vi "Scan Barcode.vi"(0 "Operator":string, 11 "error in":errorcluster) -> (4 "Operator Name Out":string, 6 "Serial Number Out":string, 8 "Cancelled?":bool, 15 "error out":errorcluster)   [LabVIEW 2024]
doc: "User inputs name and serial number to log with results. Username persists between subsequent test."
uses:
  <vilib>/addons/_JKI Toolkits/State Machine/_JKI_lib_State_Machine.llb/Select State(s)_err__jki_lib_state_machine.vi
  <vilib>/addons/_JKI Toolkits/State Machine/_JKI_lib_State_Machine.llb/Periodic Trigger__ogtk__JKI-SM__jki_lib_state_machine.vi
  <userlib>/_OpenG.lib/appcontrol/appcontrol.llb/openg_application_control.lvlib
  <userlib>/_OpenG.lib/time/time.llb/openg_time.lvlib
panel:
  in  "OK":bool
  in  "Cancel":bool
  in  "Serial Number":string
  # "SCAN BARCODE"
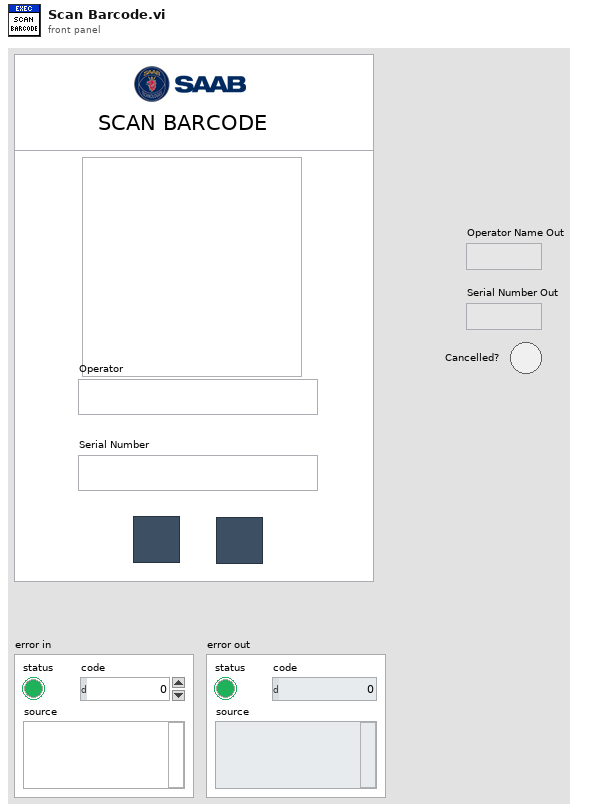
[diagram p1: front panel]
types:
  T1 = enum32{"Invalid", "Standard", "Closed", "Hidden", "Minimized", "Maximized"}
  T2 = enum32{"invalid app kind", "Development System", "Run Time System", "Student Edition", "Embedded LabVIEW", "Evaluation", "Custom"}
  T3 = cluster{"Core":cluster{"Current VI Reference":refnum<vi>, "Close Panel on Exit?":bool}, "Operator":string, "Serial Number":string}
  T4 = cluster{"Current VI Reference":refnum<vi>, "Close Panel on Exit?":bool}
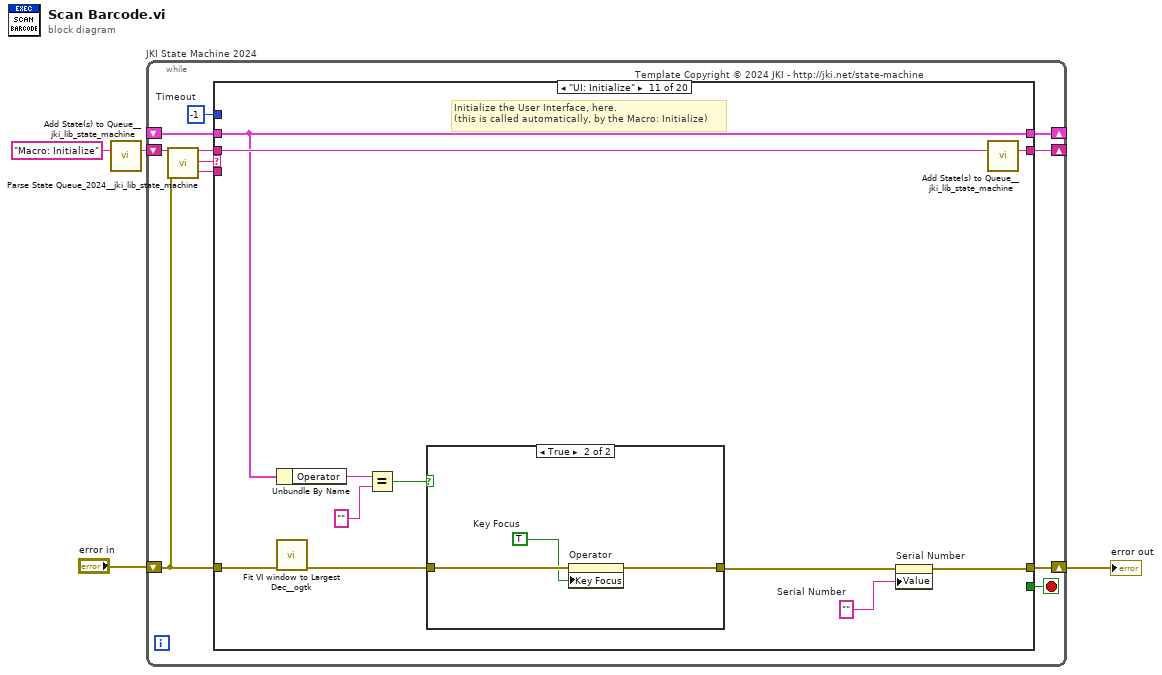
[diagram p0: block diagram]
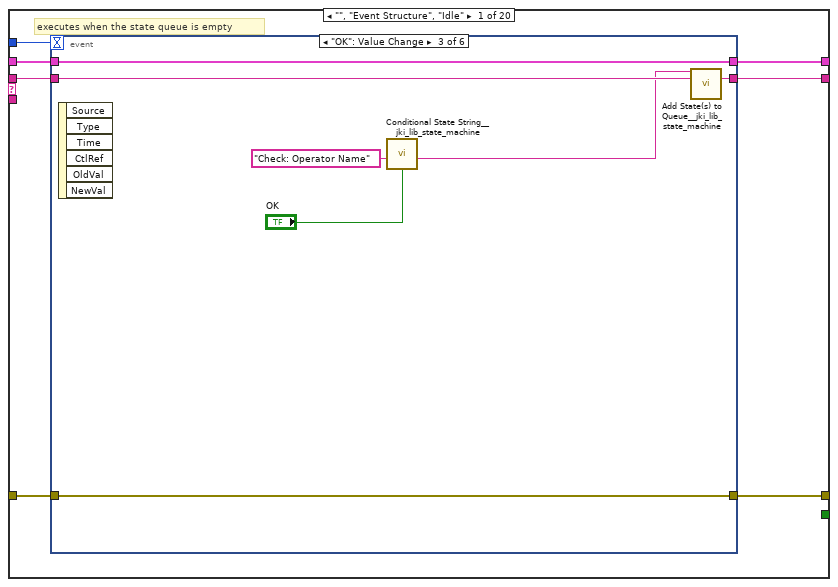
[diagram p2: hidden frame]
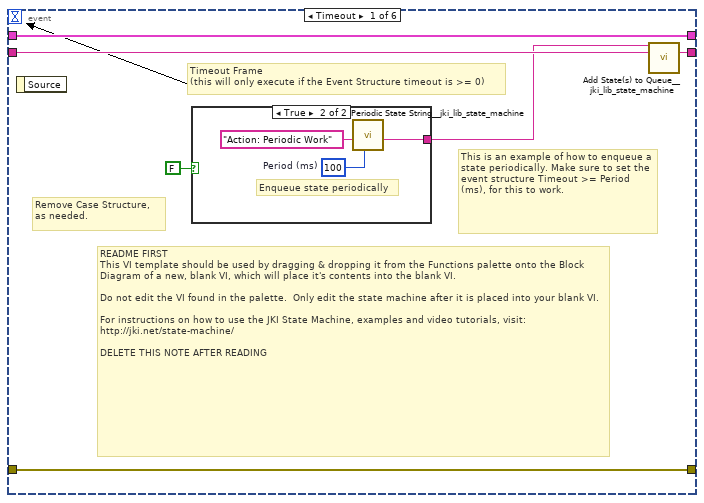
[diagram p3: hidden frame]
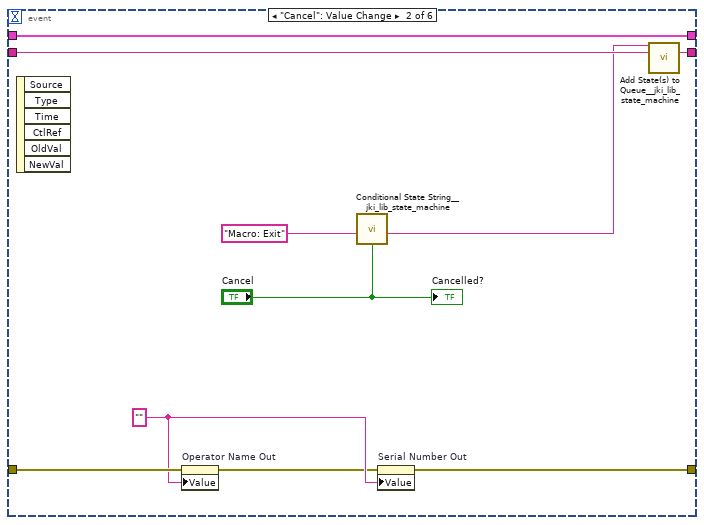
[diagram p5: hidden frame]
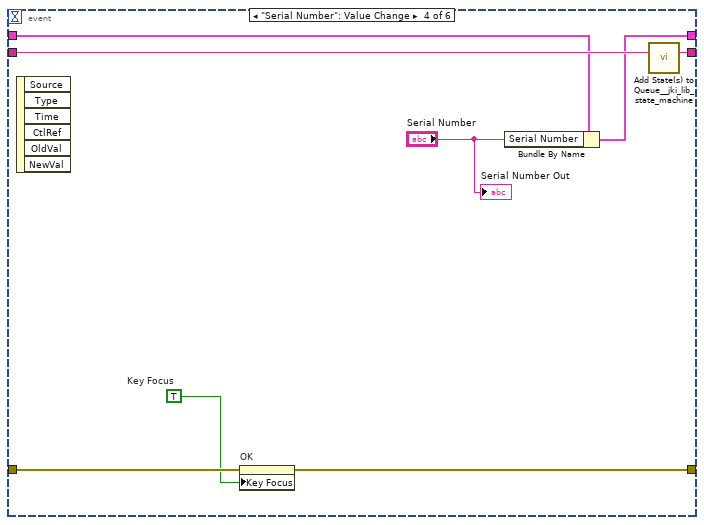
[diagram p6: hidden frame]
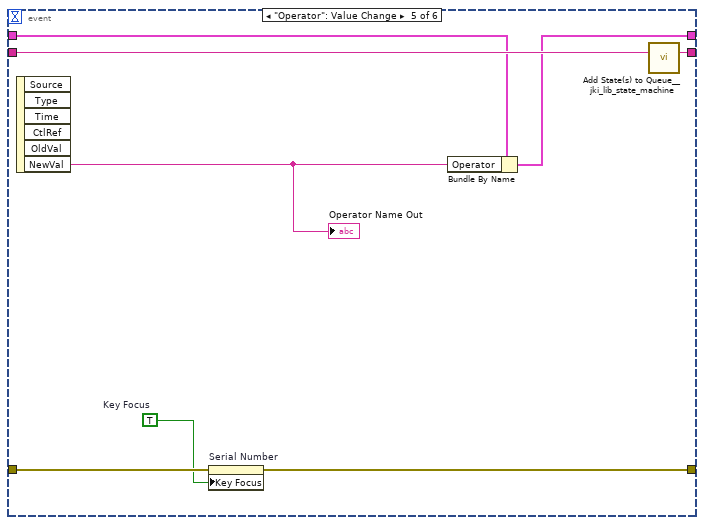
[diagram p7: hidden frame]
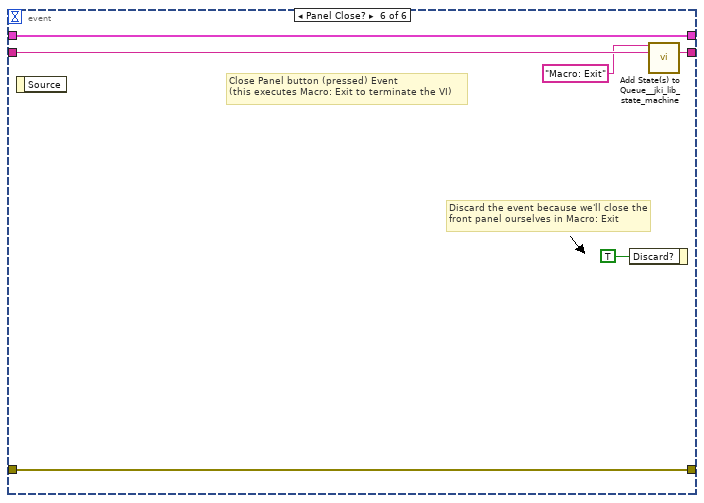
[diagram p8: hidden frame]
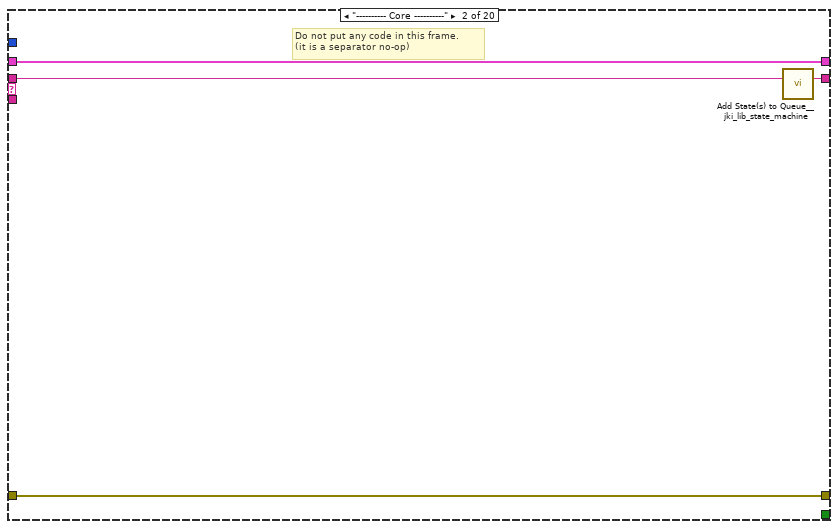
[diagram p9: hidden frame]
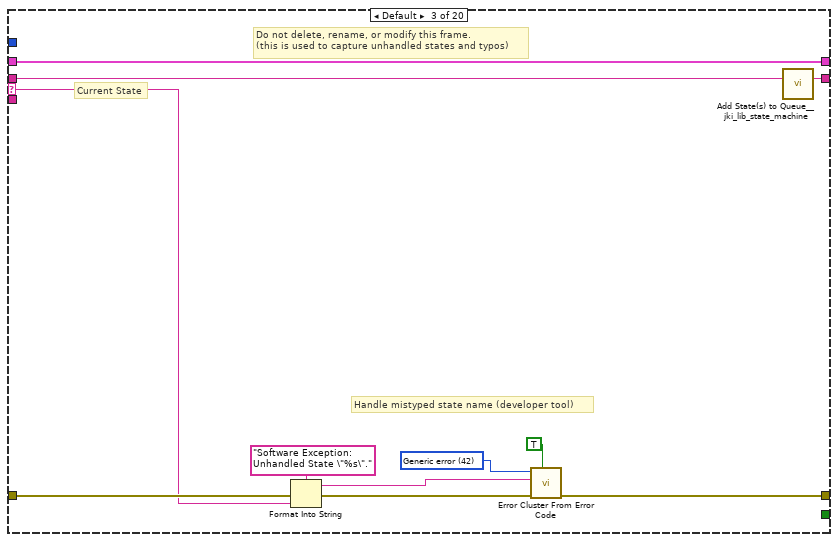
[diagram p10: hidden frame]
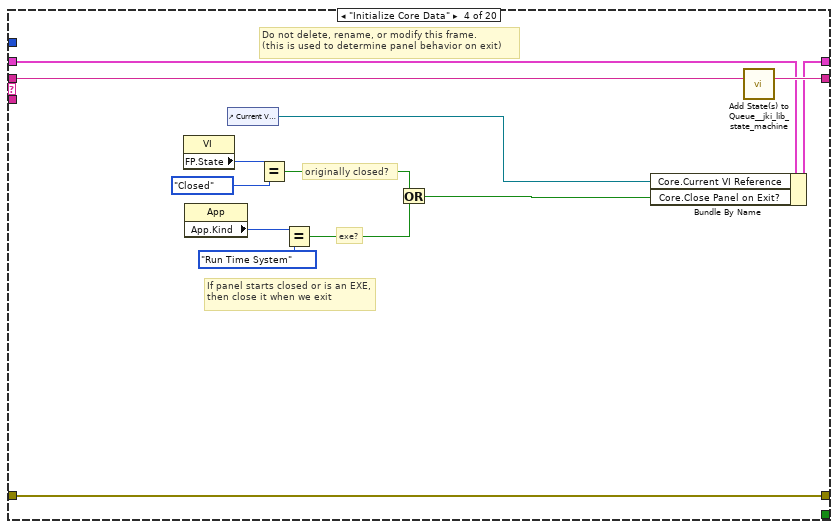
[diagram p11: hidden frame]
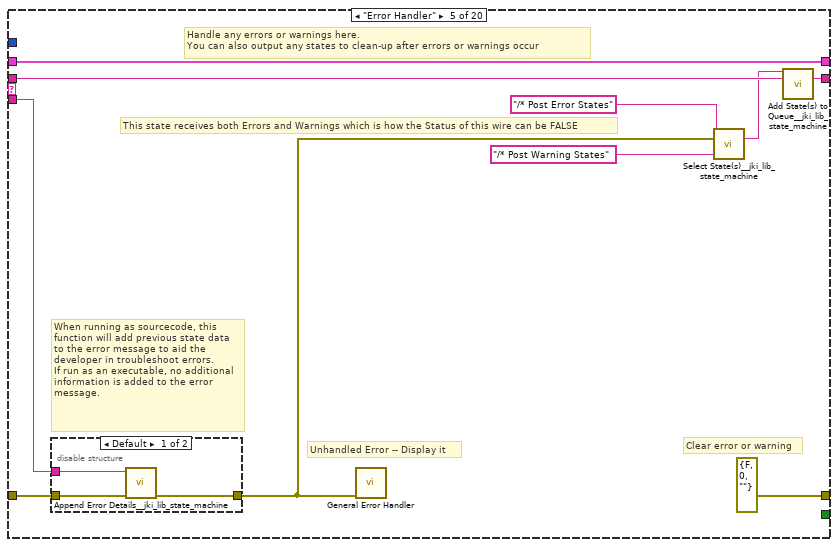
[diagram p12: hidden frame]
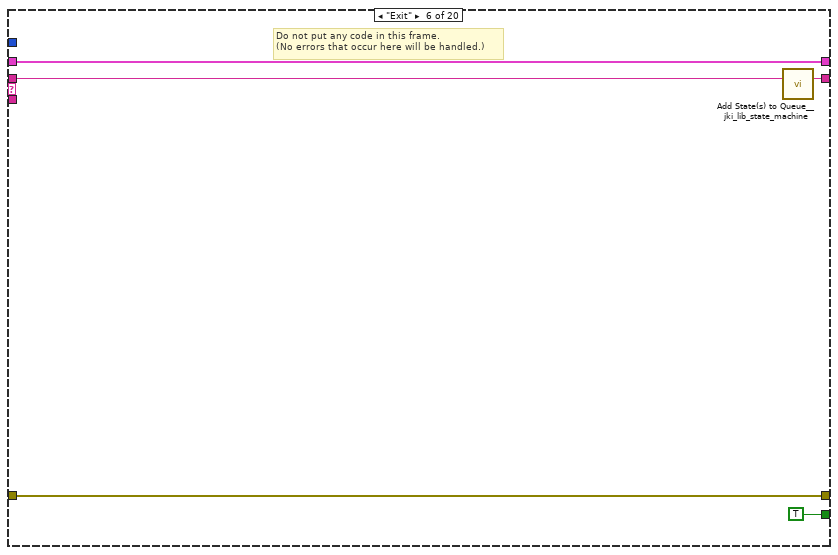
[diagram p14: hidden frame]
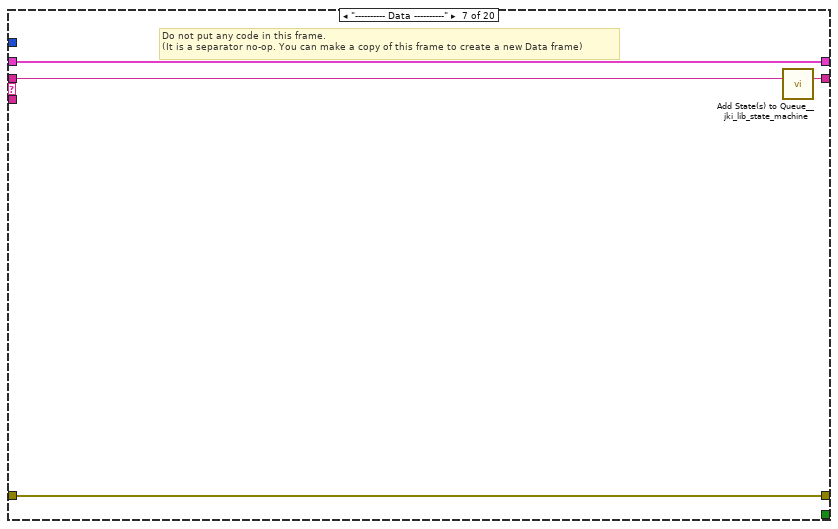
[diagram p15: hidden frame]
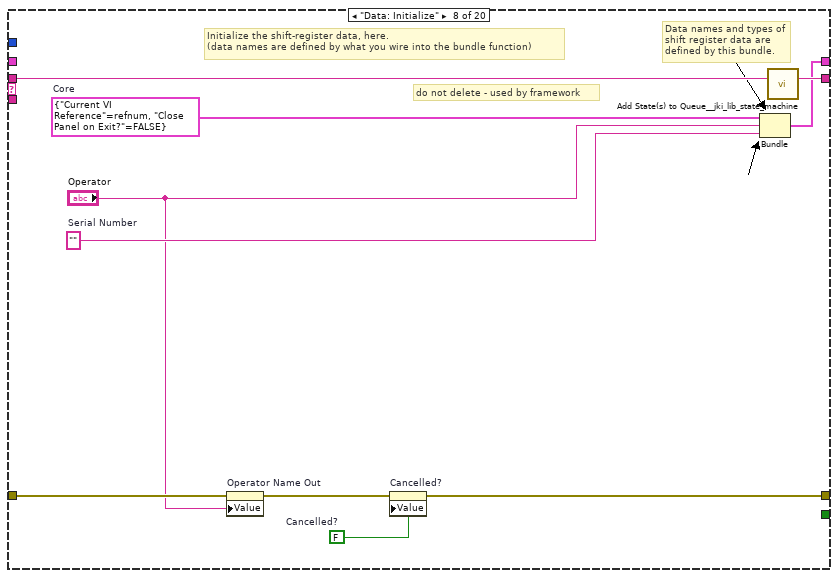
[diagram p16: hidden frame]
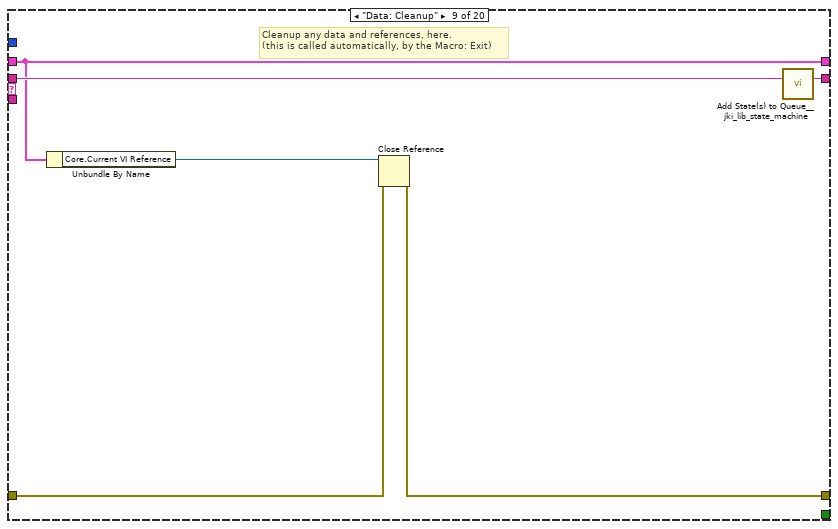
[diagram p17: hidden frame]
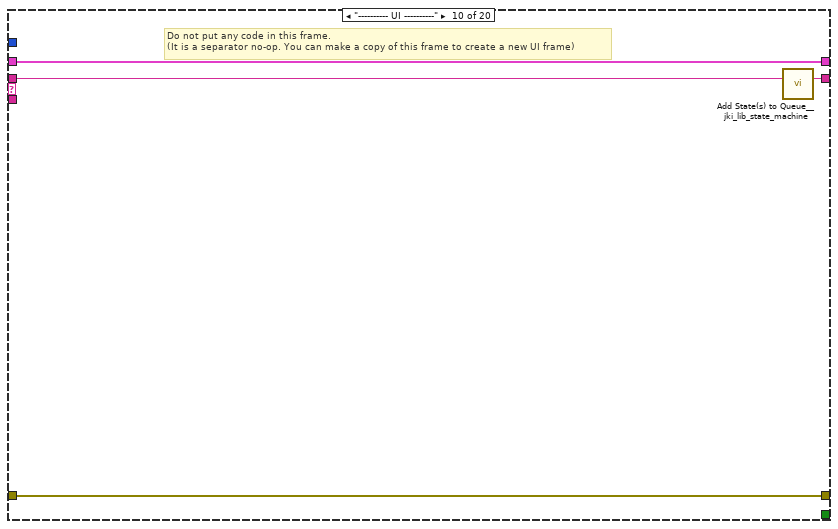
[diagram p18: hidden frame]
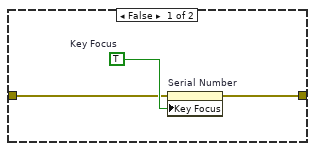
[diagram p19: hidden frame]
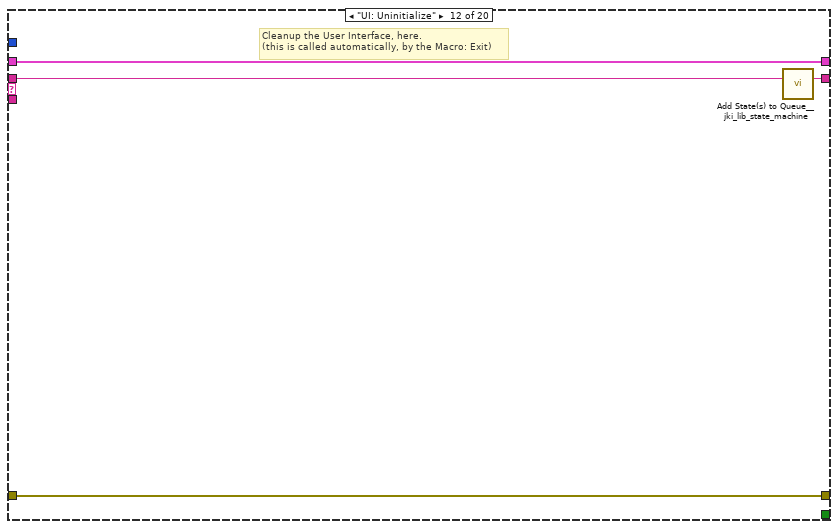
[diagram p20: hidden frame]
diagram:
  n1 = call <vilib>:"Add State(s) to Queue__jki_lib_state_machine.vi"("State(s) in (\"\")"="Macro: Initialize") -> ("States Out"=w4:string)  [unwired: 14 in]
  n2 = while "JKI State Machine 2024" {
    shift-right: [w8] -> _
    shift-left: _ -> [w7]
    shift-right: [w11] -> w1
    shift-left: "error in" -> [w5]
    shift-right: [w10] -> _
    shift-left: w4 -> [w12]
    stop <- w9 stop-if-true
    w6 = -1  # Timeout
    # "Template Copyright © 2024 JKI - http://jki.net/state-machine"
    n3 = call <vilib>:"Parse State Queue_2024__jki_lib_state_machine.vi"("State Queue"=w12, "Error In (no error)"=w5) -> ("Remaining States"=w14:string, "Current State"=w15:string, "Arguments"=w13:string)  [unwired: 11 in]
    n4 = case shown="\"UI: Initialize\"" w15 {
      selector: w15 -> [_ _ w75 _ _ _ _ _ _ _ _ _ _ _ _ _ _ _ _ _]
      tunnel: w14 -> [w22 w74 w79 w98 w108 w117 w121 w131 w137 w141 w152 w162 w168 w179 w248 w253 w262 w266 w275 w297]
      tunnel: w13 -> [_ _ _ _ w103 _ _ _ _ _ _ _ w163 w173 _ _ _ _ _ _]
      tunnel: w7 -> [w20 w71 w77 w91 w105 w115 w118 _ w132 w138 w148 w160 w166 w175 w245 w250 w260 w263 w269 w290]
      tunnel: [w19 w72 w81 w95 errorcluster {"status"=FALSE, "code"=0, "source"=""} ("error out") w114 w119 w123 w133 w139 w144 w159 w164 w176 w246 w251 w257 w264 w267 w291] -> w11
      tunnel: w5 -> [w16 w72 w80 w95 w104 w114 w119 w126 w134 w139 w149 w159 w165 w177 w246 w251 w257 w264 w270 w292]
      tunnel: [w21 w73 w78 w97 w107 w116 w120 w130 w136 w140 w151 w161 w167 w178 w247 w252 w261 w265 w274 w296] -> w10
      tunnel: [_ _ _ _ _ TRUE _ _ _ _ _ _ _ _ _ _ _ _ _ _] -> w9
      tunnel: [w18 w71 w77 w96 w105 w115 w118 w129 w132 w138 w148 w160 w166 w175 w245 w250 w260 w263 w269 w290] -> w8
      tunnel: w6 -> [w17 _ _ _ _ _ _ _ _ _ _ _ _ _ _ _ _ _ _ _]
      frame "", "Event Structure", "Idle" {
        # "executes when the state queue is empty"
        n5 = event shown="[2] \"OK\": Value Change" {
          selector: _ -> [_ _ _ _ _ _]
          dyn-events: _ -> [_ _ _ _ _ _]
          timeout: w17 -> [_ _ _ _ _ _]
          tunnel: w22 -> [w28 w41 w48 w56 w64 w70]
          tunnel: [w27 w40 w47 w55 w63 w69] -> w21
          tunnel: w20 -> [w25 w36 w45 w54 w62 w67]
          tunnel: [w26 w32 w46 w50 w59 w68] -> w19
          tunnel: w16 -> [w26 w35 w46 w51 w58 w68]
          tunnel: [w25 w36 w45 w53 w61 w67] -> w18
          event Timeout {
            # "Remove Case Structure, as needed."
            # "This is an example of how to enqueue a state periodically. Make sure to set the event structure Timeout >= Period (ms), for this to work."
            # "README FIRST\nThis VI template should be used by dragging & dropping it from the Functions palette onto the Block Diagram of a new, blank VI, which will place it's contents into the blank VI.\n\nDo not edit the VI found in the palette.  Only edit the state machine after it is placed into your blank VI.\n\nFor instructions on how to use the JKI State Machine, examples and video tutorials, visit:\nhttp://jki.net/state-machine/\n\nDELETE THIS NOTE AFTER READING"
            # "Timeout Frame\n(this will only execute if the Event Structure timeout is >= 0)"
            n6 = event-data() -> ()  [unwired: 1 in, 1 out]
            n7 = case shown="True" FALSE {
              tunnel: [_ w31] -> w24
              frame False {
              }
              frame True {
                w29 = u32 100  # Period (ms)
                # "Enqueue state periodically"
                n8 = call <vilib>:"Periodic State String__jki_lib_state_machine.vi"("Period (ms)"=w29, "State"="Action: Periodic Work") -> ("State Out"=w31:string)  [unwired: 9 in]
              }
            }
            n9 = call <vilib>:"Add State(s) to Queue__jki_lib_state_machine.vi"("State(s) in Front (\"\")"=w24, "State(s) in (\"\")"=w28) -> ("States Out"=w27:string)  [unwired: 13 in]
          }
          event "Cancel": Value Change {
            w34 = ""
            n10 = event-data() -> ()  [unwired: 1 in, 6 out]
            n11 = property on="Operator Name Out" class="Str"(error in=w35, "Value"=w34) -> (error out=w33:errorcluster)  [unwired: 1 in, 1 out]
            n12 = call <vilib>:"Conditional State String__jki_lib_state_machine.vi"("Do State(s)?"="Cancel", "State"="Macro: Exit") -> ("State Out"=w38:string)  [unwired: 7 in]
            n13 = property on="Serial Number Out" class="Str"(error in=w33, "Value"=w34) -> (error out=w32:errorcluster)  [unwired: 1 in, 1 out]
            n14 = call <vilib>:"Add State(s) to Queue__jki_lib_state_machine.vi"("State(s) in Front (\"\")"=w38, "State(s) in (\"\")"=w41) -> ("States Out"=w40:string)  [unwired: 13 in]
            "Cancelled?" <- "Cancel"
          }
          event "OK": Value Change {
            n15 = event-data() -> ()  [unwired: 1 in, 6 out]
            n16 = call <vilib>:"Conditional State String__jki_lib_state_machine.vi"("Do State(s)?"="OK", "State"="Check: Operator Name") -> ("State Out"=w43:string)  [unwired: 7 in]
            n17 = call <vilib>:"Add State(s) to Queue__jki_lib_state_machine.vi"("State(s) in Front (\"\")"=w43, "State(s) in (\"\")"=w48) -> ("States Out"=w47:string)  [unwired: 13 in]
          }
          event "Serial Number": Value Change {
            w49 = TRUE  # Key Focus
            n18 = event-data() -> ()  [unwired: 1 in, 6 out]
            n19 = property on="OK" class="Bool"(error in=w51, "Key Focus"=w49) -> (error out=w50:errorcluster)  [unwired: 1 in, 1 out]
            n20 = Bundle By Name(cluster=w54, "Serial Number"="Serial Number") -> (w53:T3)
            n21 = call <vilib>:"Add State(s) to Queue__jki_lib_state_machine.vi"("State(s) in (\"\")"=w56) -> ("States Out"=w55:string)  [unwired: 14 in]
            "Serial Number Out" <- "Serial Number"
          }
          event "Operator": Value Change {
            w57 = TRUE  # Key Focus
            n22 = event-data() -> ("NewVal"=w60:string)  [unwired: 1 in, 5 out]
            "Operator Name Out" <- w60
            n23 = property on="Serial Number" class="Str"(error in=w58, "Key Focus"=w57) -> (error out=w59:errorcluster)  [unwired: 1 in, 1 out]
            n24 = Bundle By Name(cluster=w62, "Operator"=w60) -> (w61:T3)
            n25 = call <vilib>:"Add State(s) to Queue__jki_lib_state_machine.vi"("State(s) in (\"\")"=w64) -> ("States Out"=w63:string)  [unwired: 14 in]
          }
          event Panel Close? {
            # "Discard the event because we'll close the front panel ourselves in Macro: Exit"
            # "Close Panel button (pressed) Event\n(this executes Macro: Exit to terminate the VI)"
            n26 = event-data() -> ()  [unwired: 1 in, 1 out]
            n27 = event-data("Discard?"=TRUE) -> ()  [unwired: 1 in, 1 out]
            n28 = call <vilib>:"Add State(s) to Queue__jki_lib_state_machine.vi"("State(s) in Front (\"\")"="Macro: Exit", "State(s) in (\"\")"=w70) -> ("States Out"=w69:string)  [unwired: 13 in]
          }
        }
      }
      frame "---------- Core ----------" {
        # "Do not put any code in this frame.\n(it is a separator no-op)"
        n29 = call <vilib>:"Add State(s) to Queue__jki_lib_state_machine.vi"("State(s) in (\"\")"=w74) -> ("States Out"=w73:string)  [unwired: 14 in]
      }
      frame Default {
        w84 = 42 items=["No error", "Argument error", "Memory is full", "Out of zone", "End of file", "File already open", "Generic file I/O error", "File not found", "File permission error", "Disk is full", "Duplicate path", "Too many files open", "System feature not enabled", "Resource file not found", "Cannot add resource", "Resource not found", "Image not found", "Image memory error", "Pen does not exist", "Config type invalid", "Config token not found", "Config parse error", "Config memory error", "Bad external code format", "Bad external code offset", "External code not present", "Null window", "Destroy window error", "Null menu", "Print aborted", "Bad print record", "Print driver error", "Windows error during printing", "Memory error during printing", "Print dialog error", "Generic print error", "Invalid device refnum", "Device not found", "Device parameter error", "Device unit error", "Cannot open device", "Device call aborted", "Generic error", "Cancelled by user", "Object ID too low", "Object ID too high", "Object not in heap", "Unknown heap", "Unknown object (invalid DefProc)", "Unknown object (DefProc not in table)", "Message out of range", "Invalid (null) method", "Unknown message", "Manager call not supported", "Bad address", "Network operation in progress", "Network operation timed out", "Connection is busy", "Network attribute not supported", "Network error", "Address in use", "System out of memory", "Connection aborted", "Connection refused", "Not connected", "Already connected", "Connection closed", "Initialization error (interapplication manager)", "Bad occurrence", "Wait on unbound occurrence handler", "Occurrence queue overflow", "Datalog type conflict", "Unused", "Unrecognized type (interapplication manager)", "Memory corrupt", "Failed to make temporary DLL", "Old CIN version", "Drag socket not found", "Failed to load drop-object", "Failed to register OLE object", "Failed to release OLE object", "Format specifier type mismatch", "Unknown format specifier", "Too few format specifiers", "Too many format specifiers", "Scan failed", "Newer CIN version", "Error converting to variant", "Runtime menu error", "Password tampered", "Variant attribute not found", "Incompatible variant data type", "Event data is not available", "Event Store is not present", "Occurrence is not found", "Event Queue is not created", "Event info is not available", "Refnum passed is NULL", "Error retrieving Class GUID", "Error retrieving CoClass GUID", "Error retrieving TypeLib GUID.", "Bad built application magic bytes.", "Specific driver is different from the specific driver associated with the Logical Name.", "There is no session opened to the class driver.", "Max Error", "MAX - Error with config objects", "MAX - Error loading configuration", "MAX - Group not supported"]
        # "Current State"
        # "Do not delete, rename, or modify this frame.\n(this is used to capture unhandled states and typos)"
        # "Handle mistyped state name (developer tool)"
        n30 = Format Into String(format string="Software Exception: Unhandled State \"%s\"." ("message"), error in=w80, w75) -> (resulting string=w83:string, error out=w82:errorcluster)  [unwired: 1 in]
        n31 = call <vilib>:"Error Cluster From Error Code.vi"("show call chain? (False)"=TRUE, "error in (no error)"=w82, "error message (\"\")"=w83, "error code (0)"=w84) -> ("error out"=w81:errorcluster)  [unwired: 5 in]
        n32 = call <vilib>:"Add State(s) to Queue__jki_lib_state_machine.vi"("State(s) in (\"\")"=w79) -> ("States Out"=w78:string)  [unwired: 14 in]
      }
      frame "Initialize Core Data" {
        # "Do not delete, rename, or modify this frame.\n(this is used to determine panel behavior on exit)"
        # "originally closed?"
        # "exe?"
        # "If panel starts closed or is an EXE, then close it when we exit"
        n33 = property class="VI"() -> ("FP.State"=w88:T1)  [unwired: 2 in, 2 out]
        n34 = property class="App"() -> ("App.Kind"=w94:T2)  [unwired: 2 in, 2 out]
        n35 = control-ref of="Current VI Reference"() -> (w89:refnum<vi>)
        n36 = Equal?(x=w88, y=T1."Closed" ("Front Panel Window:State")) -> (x = y?=w86:bool)
        n37 = Equal?(x=w94, y=T2."Run Time System" ("Application:Kind")) -> (x = y?=w92:bool)
        n38 = Or(x=w86, y=w92) -> (x .or. y?=w90:bool)
        n39 = Bundle By Name(cluster=w91, "Core.Current VI Reference"=w89, "Core.Close Panel on Exit?"=w90) -> (w96:T3)
        n40 = call <vilib>:"Add State(s) to Queue__jki_lib_state_machine.vi"("State(s) in (\"\")"=w98) -> ("States Out"=w97:string)  [unwired: 14 in]
      }
      frame "Error Handler" {
        # "When running as sourcecode, this function will add previous state data to the error message to aid the developer in troubleshoot errors.\nIf run as an executable, no additional information is added to the error message."
        # "This state receives both Errors and Warnings which is how the Status of this wire can be FALSE"
        # "Unhandled Error -- Display it"
        # "Handle any errors or warnings here.\nYou can also output any states to clean-up after errors or warnings occur"
        # "Clear error or warning"
        n41 = disable-structure shown="Default" {
          disable-tunnel: w104 -> [w111 w112]
          disable-tunnel: w103 -> [w110 _]
          disable-tunnel: [w109 w112] -> w102
          frame condition #0 (active) {
            n42 = call <vilib>:"Append Error Details__jki_lib_state_machine.vi"("error in (no error)"=w111, "Previous State and Argument(s)"=w110) -> ("error out"=w109:errorcluster)  [unwired: 9 in]
          }
          frame condition #1 {
          }
        }
        n43 = call <vilib>:"General Error Handler.vi"("error in (no error)"=w102) -> ()  [unwired: 10 in, 5 out]
        n44 = call-poly <vilib>:"Select State(s)__jki_lib_state_machine.vi"("State(s) if True (\"\")"="/* Post Error States", "Select"=w102, "State(s) if False (\"\")"="/* Post Warning States") -> ("States Out"=w100:string)  [unwired: 12 in]
        n45 = call <vilib>:"Add State(s) to Queue__jki_lib_state_machine.vi"("State(s) in Front (\"\")"=w100, "State(s) in (\"\")"=w108) -> ("States Out"=w107:string)  [unwired: 13 in]
      }
      frame "Exit" {
        # "Do not put any code in this frame.\n(No errors that occur here will be handled.)"
        n46 = call <vilib>:"Add State(s) to Queue__jki_lib_state_machine.vi"("State(s) in (\"\")"=w117) -> ("States Out"=w116:string)  [unwired: 14 in]
      }
      frame "---------- Data ----------" {
        # "Do not put any code in this frame.\n(It is a separator no-op. You can make a copy of this frame to create a new Data frame)"
        n47 = call <vilib>:"Add State(s) to Queue__jki_lib_state_machine.vi"("State(s) in (\"\")"=w121) -> ("States Out"=w120:string)  [unwired: 14 in]
      }
      frame "Data: Initialize" {
        w122 = FALSE  # Cancelled?
        w127 = T4 {"Current VI Reference"=refnum, "Close Panel on Exit?"=FALSE}  # Core
        w128 = ""  # Serial Number
        # "do not delete - used by framework"
        # "Data names and types of shift register data are defined by this bundle."
        # "Initialize the shift-register data, here.\n(data names are defined by what you wire into the bundle function)"
        n48 = property on="Operator Name Out" class="Str"(error in=w126, "Value"="Operator") -> (error out=w124:errorcluster)  [unwired: 1 in, 1 out]
        n49 = property on="Cancelled?" class="Bool (strict)"(error in=w124, "Value"=w122) -> (error out=w123:errorcluster)  [unwired: 1 in, 1 out]
        n50 = Bundle("Core"=w127, "Operator"="Operator", "Serial Number"=w128) -> (w129:T3)  [unwired: 1 in]
        n51 = call <vilib>:"Add State(s) to Queue__jki_lib_state_machine.vi"("State(s) in (\"\")"=w131) -> ("States Out"=w130:string)  [unwired: 14 in]
      }
      frame "Data: Cleanup" {
        # "Cleanup any data and references, here.\n(this is called automatically, by the Macro: Exit)"
        n52 = Unbundle By Name(w132) -> ("Core.Current VI Reference"=w135:refnum<vi>)
        n53 = Close Reference(reference=w135, error in (no error)=w134) -> (error out=w133:errorcluster)
        n54 = call <vilib>:"Add State(s) to Queue__jki_lib_state_machine.vi"("State(s) in (\"\")"=w137) -> ("States Out"=w136:string)  [unwired: 14 in]
      }
      frame "---------- UI ----------" {
        # "Do not put any code in this frame.\n(It is a separator no-op. You can make a copy of this frame to create a new UI frame)"
        n55 = call <vilib>:"Add State(s) to Queue__jki_lib_state_machine.vi"("State(s) in (\"\")"=w141) -> ("States Out"=w140:string)  [unwired: 14 in]
      }
      frame "UI: Initialize" {
        w142 = ""  # Serial Number
        # "Initialize the User Interface, here.\n(this is called automatically, by the Macro: Initialize)"
        n56 = Unbundle By Name(w148) -> ("Operator"=w147:string)
        n57 = call <userlib>:"Fit VI window to Largest Dec__ogtk.vi"("error in (no error)"=w149) -> ("error out"=w150:errorcluster)  [unwired: 5 in, 1 out]
        n58 = Equal?(x=w147, y="") -> (x = y?=w145:bool)
        n59 = case shown="True" w145 {
          tunnel: [w154 w157] -> w143
          tunnel: w150 -> [w153 w158]
          frame False {
            w155 = TRUE  # Key Focus
            n60 = property on="Serial Number" class="Str"(error in=w153, "Key Focus"=w155) -> (error out=w154:errorcluster)  [unwired: 1 in, 1 out]
          }
          frame True {
            w156 = TRUE  # Key Focus
            n61 = property on="Operator" class="Str"(error in=w158, "Key Focus"=w156) -> (error out=w157:errorcluster)  [unwired: 1 in, 1 out]
          }
        }
        n62 = property on="Serial Number" class="Str"(error in=w143, "Value"=w142) -> (error out=w144:errorcluster)  [unwired: 1 in, 1 out]
        n63 = call <vilib>:"Add State(s) to Queue__jki_lib_state_machine.vi"("State(s) in (\"\")"=w152) -> ("States Out"=w151:string)  [unwired: 14 in]
      }
      frame "UI: Uninitialize" {
        # "Cleanup the User Interface, here.\n(this is called automatically, by the Macro: Exit)"
        n64 = call <vilib>:"Add State(s) to Queue__jki_lib_state_machine.vi"("State(s) in (\"\")"=w162) -> ("States Out"=w161:string)  [unwired: 14 in]
      }
      frame "UI: Cursor Set" {
        # "Argument"
        # "Set and Unset Cursor Busy.\n(Usage: \"UI: Cursor Set >> Busy|Idle\")"
        n65 = case shown="\"Idle\", Default" w163 {
          tunnel: w165 -> [w170 w172]
          tunnel: [w169 w171] -> w164
          frame "Idle", Default {
            n66 = call <vilib>:"Unset Busy.vi"("error in (no error)"=w170) -> ("error out"=w169:errorcluster)  [unwired: 10 in]
          }
          frame "Busy" {
            n67 = call <vilib>:"Set Busy.vi"("error in (no error)"=w172) -> ("error out"=w171:errorcluster)  [unwired: 9 in, 1 out]
          }
        }
        n68 = call <vilib>:"Add State(s) to Queue__jki_lib_state_machine.vi"("State(s) in (\"\")"=w168) -> ("States Out"=w167:string)  [unwired: 14 in]
      }
      frame "UI: Front Panel State" {
        # "Argument"
        # "Set Front Panel Open or Closed\n(Usage: \"UI: Front Panel State >> Open|Close\")"
        n69 = Unbundle By Name(w175) -> ("Core.Current VI Reference"=w174:refnum<vi>)
        n70 = case shown="\"Minimize\", \"Minimized\"" w173 {
          tunnel: w177 -> [w185 w200 w211 w224 w237]
          tunnel: [w187 w201 w213 w226 w239] -> w176
          tunnel: w174 -> [w186 w198 w212 w225 w238]
          frame "Open", "Standard", Default {
            w180 = T1."Standard" ("State")
            n71 = property class="VI"(reference=w186, error in=w185) -> (reference out=w183:refnum<vi>, error out=w184:errorcluster, "FP.State"=w182:T1)
            n72 = Not Equal?(x=w182, y=w180) -> (x != y?=w181:bool)
            n73 = case shown="True" w181 {
              tunnel: [w191 w193] -> w187
              tunnel: w184 -> [w190 w193]
              tunnel: w183 -> [w189 _]
              tunnel: w180 -> [w188 _]
              frame True {
                n74 = invoke class="VI" method="FP.Open"(reference=w189, error in=w190, "Activate"=TRUE, "State"=w188) -> (error out=w191:errorcluster)  [unwired: 1 in, 4 out]
              }
              frame False {
              }
            }
          }
          frame "Close", "Closed" {
            n75 = property class="VI"(reference=w198, error in=w200) -> (reference out=w197:refnum<vi>, error out=w199:errorcluster, "FP.State"=w195:T1)
            n76 = Not Equal?(x=w195, y=T1."Closed" ("Front Panel Window:State")) -> (x != y?=w194:bool)
            n77 = case shown="True" w194 {
              tunnel: [w202 w205] -> w201
              tunnel: w199 -> [w202 w204]
              tunnel: w197 -> [_ w203]
              frame False {
              }
              frame True {
                n78 = invoke class="VI" method="FP.Close"(reference=w203, error in=w204) -> (error out=w205:errorcluster)  [unwired: 1 in, 2 out]
              }
            }
          }
          frame "Hidden", "Hide" {
            w206 = T1."Hidden" ("State")
            n79 = property class="VI"(reference=w212, error in=w211) -> (reference out=w209:refnum<vi>, error out=w210:errorcluster, "FP.State"=w208:T1)
            n80 = Not Equal?(x=w208, y=w206) -> (x != y?=w207:bool)
            n81 = case shown="True" w207 {
              tunnel: [w217 w218] -> w213
              tunnel: w210 -> [w216 w218]
              tunnel: w209 -> [w215 _]
              tunnel: w206 -> [w214 _]
              frame True {
                n82 = invoke class="VI" method="FP.Open"(reference=w215, error in=w216, "State"=w214) -> (error out=w217:errorcluster)  [unwired: 2 in, 4 out]
              }
              frame False {
              }
            }
          }
          frame "Minimize", "Minimized" {
            w219 = T1."Minimized" ("State")
            n83 = property class="VI"(reference=w225, error in=w224) -> (reference out=w222:refnum<vi>, error out=w223:errorcluster, "FP.State"=w221:T1)
            n84 = Not Equal?(x=w221, y=w219) -> (x != y?=w220:bool)
            n85 = case shown="True" w220 {
              tunnel: [w230 w231] -> w226
              tunnel: w223 -> [w229 w231]
              tunnel: w222 -> [w228 _]
              tunnel: w219 -> [w227 _]
              frame True {
                n86 = invoke class="VI" method="FP.Open"(reference=w228, error in=w229, "State"=w227) -> (error out=w230:errorcluster)  [unwired: 2 in, 4 out]
              }
              frame False {
              }
            }
          }
          frame "Maximize", "Maximized" {
            w232 = T1."Maximized" ("State")
            n87 = property class="VI"(reference=w238, error in=w237) -> (reference out=w235:refnum<vi>, error out=w236:errorcluster, "FP.State"=w234:T1)
            n88 = Not Equal?(x=w234, y=w232) -> (x != y?=w233:bool)
            n89 = case shown="True" w233 {
              tunnel: [w243 w244] -> w239
              tunnel: w236 -> [w242 w244]
              tunnel: w235 -> [w241 _]
              tunnel: w232 -> [w240 _]
              frame True {
                n90 = invoke class="VI" method="FP.Open"(reference=w241, error in=w242, "State"=w240) -> (error out=w243:errorcluster)  [unwired: 2 in, 4 out]
              }
              frame False {
              }
            }
          }
        }
        n91 = call <vilib>:"Add State(s) to Queue__jki_lib_state_machine.vi"("State(s) in (\"\")"=w179) -> ("States Out"=w178:string)  [unwired: 14 in]
      }
      frame "---------- Macro ----------" {
        # "Do not put any code in this frame.\n(It is a separator no-op. You can make a copy of this frame to create a new Macro frame)"
        n92 = call <vilib>:"Add State(s) to Queue__jki_lib_state_machine.vi"("State(s) in (\"\")"=w248) -> ("States Out"=w247:string)  [unwired: 14 in]
      }
      frame "Macro: Initialize" {
        w249 = "Data: Initialize\nInitialize Core Data\nUI: Initialize\nUI: Front Panel State >> Open"  # Data: Initialize Initialize Core Data UI: Initialize UI: Front Panel State >> Open
        # "Initialization Macro\n(This is called once, when the VI starts)"
        n93 = call <vilib>:"Add State(s) to Queue__jki_lib_state_machine.vi"("State(s) in Front (\"\")"=w249, "State(s) in (\"\")"=w253) -> ("States Out"=w252:string)  [unwired: 13 in]
      }
      frame "Macro: Exit" {
        # "Exit Macro\n(This is called once, when the VI exits)"
        n94 = Unbundle By Name(w260) -> ("Core.Close Panel on Exit?"=w255:bool)
        n95 = call <vilib>:"Conditional State String__jki_lib_state_machine.vi"("Do State(s)?"=w255, "State"="UI: Front Panel State >> Close") -> ("State Out"=w254:string)  [unwired: 7 in]
        n96 = call <vilib>:"Add State(s) to Queue__jki_lib_state_machine.vi"("State(s) in (\"\")"=w254, "State(s) at Back (\"\")"="UI: Uninitialize\nData: Cleanup\nExit") -> ("States Out"=w258:string)  [unwired: 13 in]
        n97 = call <vilib>:"Add State(s) to Queue__jki_lib_state_machine.vi"("State(s) in Front (\"\")"=w258, "State(s) in (\"\")"=w262) -> ("States Out"=w261:string)  [unwired: 13 in]
      }
      frame "---------- Check ----------" {
        # "Template Separator\n(You can make a copy of, or modify, this frame)"
        n98 = call <vilib>:"Add State(s) to Queue__jki_lib_state_machine.vi"("State(s) in (\"\")"=w266) -> ("States Out"=w265:string)  [unwired: 14 in]
      }
      frame "Check: Operator Name" {
        n99 = Unbundle By Name(w269) -> ("Operator"=w273:string)
        n100 = Equal?(x=w273, y="") -> (x = y?=w271:bool)
        n101 = case shown="True" w271 {
          tunnel: w270 -> [w276 w281]
          tunnel: [w276 w278] -> w267
          tunnel: ["Check: Serial Number" ""] -> w268
          frame False {
          }
          frame True {
            n102 = flat-sequence {
              tunnel: w281 -> [w282]
              tunnel: [w282] -> w279
              tunnel: w279 -> [w285]
              tunnel: [w288] -> w278
              frame #0 {
                w283 = "Operator name field\ncannot be empty"  # message
                n103 = One Button Dialog(message=w283) -> ()  [unwired: 1 in, 1 out]
              }
              frame #1 {
                w287 = TRUE  # Key Focus
                n104 = call <userlib>:"Wait (ms)__ogtk.vi"("error in (no error)"=w285, "milliseconds to wait"=u32 10) -> ("error out"=w284:errorcluster)  [unwired: 8 in, 1 out]
                n105 = property on="Operator" class="Str"(error in=w284, "Key Focus"=w287) -> (error out=w288:errorcluster)  [unwired: 1 in, 1 out]
              }
            }
          }
        }
        n106 = call <vilib>:"Add State(s) to Queue__jki_lib_state_machine.vi"("State(s) in Front (\"\")"=w268, "State(s) in (\"\")"=w275) -> ("States Out"=w274:string)  [unwired: 13 in]
      }
      frame "Check: Serial Number" {
        n107 = Unbundle By Name(w290) -> ("Serial Number"=w295:string)
        n108 = Equal?(x=w295, y="") -> (x = y?=w293:bool)
        n109 = case shown="True" w293 {
          tunnel: w292 -> [w298 w303]
          tunnel: [w298 w300] -> w291
          tunnel: ["Macro: Exit" ""] -> w289
          frame False {
          }
          frame True {
            n110 = flat-sequence {
              tunnel: w303 -> [w304]
              tunnel: [w304] -> w301
              tunnel: w301 -> [w307]
              tunnel: [w310] -> w300
              frame #0 {
                w305 = "Serial number field\ncannot be empty"  # message
                n111 = One Button Dialog(message=w305) -> ()  [unwired: 1 in, 1 out]
              }
              frame #1 {
                w309 = TRUE  # Key Focus
                n112 = call <userlib>:"Wait (ms)__ogtk.vi"("error in (no error)"=w307, "milliseconds to wait"=u32 10) -> ("error out"=w308:errorcluster)  [unwired: 8 in, 1 out]
                n113 = property on="Serial Number" class="Str"(error in=w308, "Key Focus"=w309) -> (error out=w310:errorcluster)  [unwired: 1 in, 1 out]
              }
            }
          }
        }
        n114 = call <vilib>:"Add State(s) to Queue__jki_lib_state_machine.vi"("State(s) in Front (\"\")"=w289, "State(s) in (\"\")"=w297) -> ("States Out"=w296:string)  [unwired: 13 in]
      }
    }
  }
  "error out" <- w1
